vi "Format table.vi"(11 "Table输入":refnum<vi>) -> ()   [LabVIEW 2016]
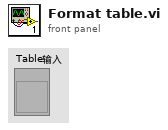
[diagram p1: front panel]
types:
  T1 = cluster{"Font Name:":string, "Size":i16, "Strikeout?":bool, "Italic?":bool, "Underline?":bool, "Outline?":bool, "Shadow?":bool, "Bold?":bool}
  T2 = enum16{"User-specified Font", "Application Font", "System Font", "Dialog Font"}
  T3 = typedef "LVFontTypeDef.ctl" = cluster{"Font Name":string, "Size":u16, "Bold":bool, "Italic":bool, "Underline":bool, "Strikeout":bool, "Color":u32}
  T4 = cluster{"left":i16, "top":i16, "right":i16, "bottom":i16}
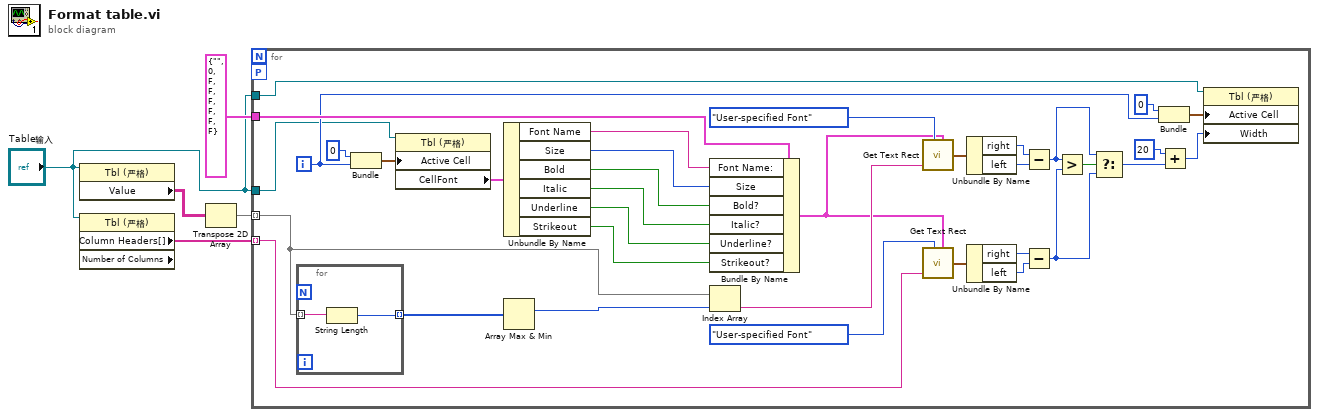
[diagram p0: block diagram]
diagram:
  n1 = property class="Tbl (严格)"(reference="Table输入") -> ("Value"=w5:string[][])  [unwired: 1 in, 2 out]
  n2 = property class="Tbl (严格)" props=["Column Headers[]", "Number of Columns"](reference="Table输入") -> ("Column Headers[]"=w1:string[])  [unwired: 1 in, 3 out]
  n3 = Transpose 2D Array(2D array=w5) -> (transposed array=w4:string[][])
  n4 = for {
    tunnel: w4 -> [w8] mode=indexing
    tunnel: T1 {"Font Name:"="", "Size"=0, "Strikeout?"=FALSE, "Italic?"=FALSE, "Underline?"=FALSE, "Outline?"=FALSE, "Shadow?"=FALSE, "Bold?"=FALSE} ("[user-specified font]") -> [w40]
    tunnel: "Table输入" -> [w34]
    tunnel: "Table输入" -> [w33]
    tunnel: w1 -> [w16] mode=indexing
    workers-P: _ -> [_]
    i -> [w39]
    n5 = for {
      tunnel: w8 -> [w42] mode=indexing
      tunnel: [w41] -> w7 mode=indexing
      n6 = String Length(string=w42) -> (length=w41:i32)
    }
    n7 = Bundle(0, w39) -> (w21:cluster{i32, i32})  [unwired: 1 in]
    n8 = property on="属性节点" class="Tbl (严格)"(reference=w34, "Active Cell"=w21) -> ("CellFont"=w22:T3)  [unwired: 1 in, 2 out]
    n9 = Unbundle By Name(w22) -> ("Font Name"=w32:string, "Size"=w31:u16, "Bold"=w30:bool, "Italic"=w29:bool, "Underline"=w28:bool, "Strikeout"=w27:bool)
    n10 = Array Max & Min(array=w7) -> (max index (indices)=w6:i32)  [unwired: 3 out]
    n11 = Bundle By Name(cluster=w40, "Font Name:"=w32, "Size"=w31, "Bold?"=w30, "Italic?"=w29, "Underline?"=w28, "Strikeout?"=w27) -> (w18:T1)
    n12 = Index Array(array=w8, index=w6) -> (element=w20:string)
    n13 = call <vilib>:"Get Text Rect.vi"("desired font(Application)"=T2."User-specified Font", "text"=w20, "[user-specified font]"=w18) -> ("rect"=w25:T4)  [unwired: 6 in]
    n14 = call <vilib>:"Get Text Rect.vi"("desired font(Application)"=T2."User-specified Font", "text"=w16, "[user-specified font]"=w18) -> ("rect"=w13:T4)  [unwired: 6 in]
    n15 = Unbundle By Name(w25) -> ("right"=w24:i16, "left"=w23:i16)
    n16 = Unbundle By Name(w13) -> ("right"=w14:i16, "left"=w15:i16)
    n17 = Subtract(x=w24, y=w23) -> (x-y=w11:i16)
    n18 = Subtract(x=w14, y=w15) -> (x-y=w10:i16)
    n19 = Greater?(x=w11, y=w10) -> (0:w12:bool)
    n20 = Select(t=w11, s=w12, f=w10) -> (s? t:f=w9:i16)
    n21 = Bundle(0, w39) -> (w35:cluster{i32, i32})  [unwired: 1 in]
    n22 = Add(x=i16 20, y=w9) -> (x+y=w36:i16)
    n23 = property on="属性节点" class="Tbl (严格)"(reference=w33, "Active Cell"=w35, "Width"=w36) -> ()  [unwired: 1 in, 2 out]
  }
